vi "PowerStatus.vi"(8 "error in (no error)":errorcluster, 11 "DAQmxTaskContainer_General in":refnum<class "DAQmxTaksContainer_General.lvclass">) -> (0 "error out":errorcluster, 2 "On/Off":bool, 3 "DAQmxTaskContainer_General out":refnum<class "DAQmxTaksContainer_General.lvclass">)   [LabVIEW 2018]
uses:
  DAQmxTaksContainer_General.lvclass
  DAQmxTaskAICurrent_General/DAQmxTaskAICurrent_General.lvclass
  DAQmxTaskAICurrent_General/DAQmxTaskAICurrent_General.lvclass/DAQmxTaskAICurrent_General.ctl
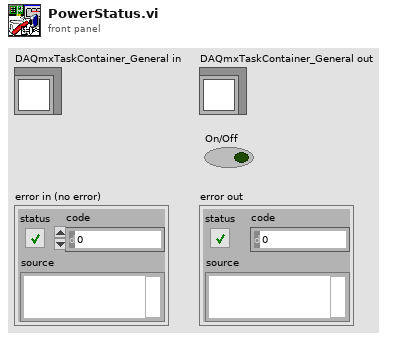
[diagram p1: front panel]
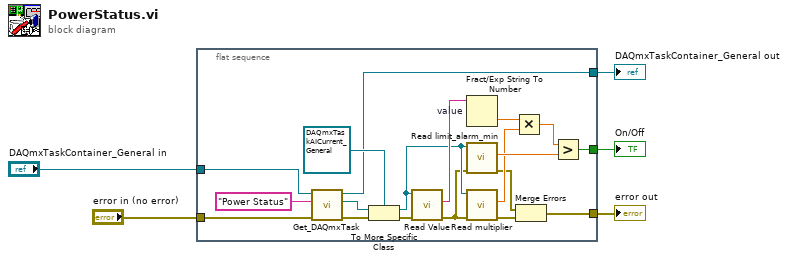
[diagram p0: block diagram]
diagram:
  n1 = flat-sequence {
    tunnel: "error in (no error)" -> [w21]
    tunnel: "DAQmxTaskContainer_General in" -> [w20]
    tunnel: [w8] -> w4
    tunnel: [w16] -> w3
    tunnel: [w6] -> w5
    frame #0 {
      n2 = call "Get_DAQmxTask.vi"("error in (no error)"=w21, "Task name"="Power Status", "DAQmxTaksContainer_General in"=w20) -> ("error out"=w18:errorcluster, "DAQmx Task"=w19:refnum<class "DAQmxTask.lvclass">, "DAQmxTaksContainer_General out"=w6:refnum<class "DAQmxTaksContainer_General.lvclass">)  [unwired: 6 in]
      n3 = To More Specific Class(target class=refnum<class "DAQmxTaskAICurrent_General.lvclass"> refnum ("DAQmxTaskAICurrent_General.lvclass"), reference=w19, error in=w18) -> (specific class reference=w15:refnum<class "DAQmxTaskAICurrent_General.lvclass">, error out=w17:errorcluster)
      n4 = call-dynamic "Read Value.vi"("error in (no error)"=w17, "DAQmxTask en entrée"=w15) -> ("error out"=w14:errorcluster, "Data string"=w23:string)  [unwired: 6 in, 2 out]
      n5 = Fract/Exp String To Number "value"(string=w23) -> (number=w13:dbl)  [unwired: 3 in, 1 out]
      n6 = call "Read limit_alarm_min.vi"("error in (no error)"=w14, "DAQmxTaskAICurrent_General in"=w15) -> ("error out"=w10:errorcluster, "limit_alarm_min"=w24:dbl)  [unwired: 7 in, 1 out]
      n7 = call "Read multiplier.vi"("error in (no error)"=w14, "DAQmxTaskAICurrent_General in"=w15) -> ("error out"=w9:errorcluster, "multiplier"=w12:dbl)  [unwired: 7 in, 1 out]
      n8 = Multiply(x=w13, y=w12) -> (x*y=w11:dbl)
      n9 = Merge Errors(w10, w9) -> (w8:errorcluster)
      n10 = Greater?(x=w11, y=w24) -> (0:w16:bool)
    }
  }
  "DAQmxTaskContainer_General out" <- w5
  "error out" <- w4
  "On/Off" <- w3
